vi "DiagCANControl.WaitForFinish.vi"(8 "error in (no error)":errorcluster, 11 "Data Value Reference in":refnum<data-value>) -> (0 "error out":errorcluster)   [LabVIEW 2019, in "Diagnostics Addon Engine.lvlib"]
uses:
  Diagnostics Addon Engine.lvlib
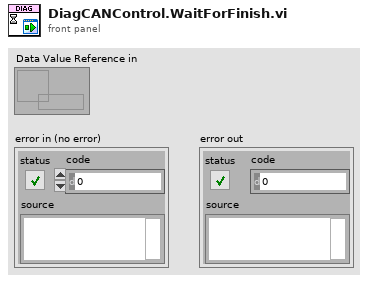
[diagram p1: front panel]
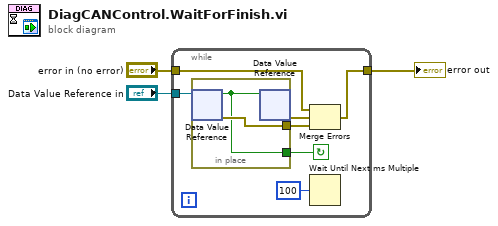
[diagram p0: block diagram]
diagram:
  n1 = while {
    tunnel: "Data Value Reference in" -> [w10]
    tunnel: "error in (no error)" -> [w4]
    tunnel: [w6] -> w1
    stop <- w9 continue-if-true
    n2 = in-place {
      in-place-border: [w12] -> w7
      in-place-border: [w11] -> w9
      n3 = in-place-dvr #1(w10) -> (w11:bool, w12:errorcluster)
      n4 = in-place-dvr #1(w11) -> (w8:errorcluster)  [unwired: 1 out]
    }
    n5 = Merge Errors(w4, w8, w7) -> (w6:errorcluster)
    n6 = Wait Until Next ms Multiple(millisecond multiple=u32 100) -> ()  [unwired: 1 out]
  }
  "error out" <- w1
